vi "Rworker.vi"(1 "Boolean":bool, 5 "IN VARIANT":variant, 7 "Name in":string, 9 "Ip":string, 11 "error in (no error)":errorcluster) -> (10 "Operation Ok":bool, 15 "error out":errorcluster)   [LabVIEW 2015]
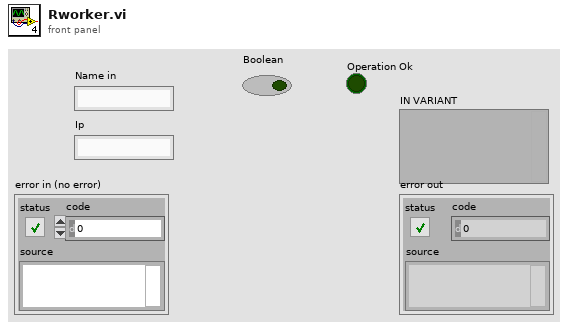
[diagram p1: front panel]
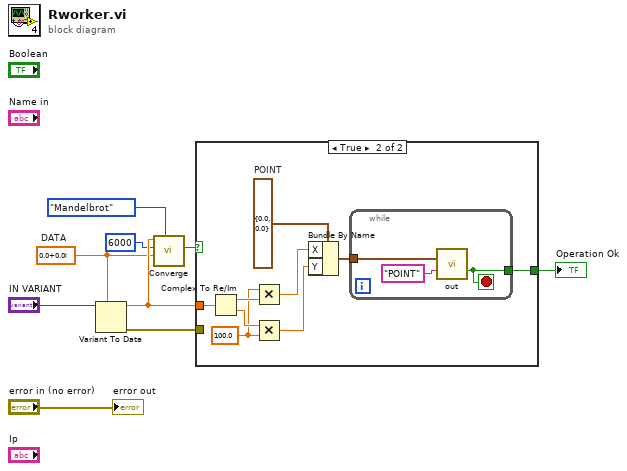
[diagram p0: block diagram]
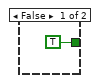
[diagram p2: hidden frame]
diagram:
  w2 = cdb 0.0+0.0i  # DATA
  n1 = Variant To Data(type=w2, Variant="IN VARIANT") -> (data=w9:cdb, error out=w8:errorcluster)  [unwired: 1 in]
  n2 = call "Converge.vi"("Fractal type"=enum16{"Mandelbrot", "Julia"}."Mandelbrot", "Z0"=w2, "Iterations"=6000, "C"=w9) -> ("IN"=w7:bool)  [unwired: 6 in, 1 out]
  n3 = case shown="True" w7 {
    tunnel: w9 -> [_ w19]
    tunnel: w8 -> [_ _]
    tunnel: [TRUE ("Operation Ok") w11] -> w4
    frame False {
    }
    frame True {
      w13 = cluster{"X":dbl, "Y":dbl} {"X"=0.0, "Y"=0.0}  # POINT
      w16 = 100.0 ("x")
      n4 = Complex To Re/Im(x + iy=w19) -> (x=w18:dbl, y=w17:dbl)
      n5 = Multiply(x=w16, y=w18) -> (x*y=w15:dbl)
      n6 = Multiply(x=w17, y=w16) -> (x*y=w14:dbl)
      n7 = Bundle By Name(cluster=w13, "X"=w15, "Y"=w14) -> (w12:cluster{"X":dbl, "Y":dbl})
      n8 = while {
        tunnel: w12 -> [w22]
        tunnel: [w21] -> w11
        stop <- w21 stop-if-true
        n9 = call "out.vi"("IN VARIANT"=w22, "Name in"="POINT" ("Name out")) -> ("Operation Ok"=w21:bool)  [unwired: 12 in, 1 out]
      }
    }
  }
  "Operation Ok" <- w4
  "error out" <- "error in (no error)"
